vi "file list from temperatures file V2.vi"(6 "monotonic segments ON/OFF":bool=TRUE, 7 "action":T4(ring)=enum."update monotonic pieces", 9 "tfolder IN":T1={"tfolder path"=path "/snowfall/Users/arcadi/Desktop/Ultrasound/Experiment/YBCO_4/Round1/Sweep12/June_2011/062511/221.16400K_300_3100_001_062511.dat", "9folder path"=path "/snowfall/Users/arcadi/Desktop/Ultrasound/Experiment/YBCO_4/Round1/Sweep12/June_2011/062511/221.16400K_300_3100_001_062511.dat", "tfolder  -  file array"=[], "from index array"=[], "timestamp array"=[]}, 11 "tfolder file path  IN":path=path "/snowfall/Users/arcadi/Desktop/Ultrasound/Experiment/YBCO_4/Round1/Sweep12/June_2011/062511/221.16400K_300_3100_001_062511.dat") -> (0 "timestamp OUT":dbl[](array[numeric]), 1 "tfolder OUT":T1={"tfolder path"=path "/snowfall/Users/arcadi/Desktop/Ultrasound/Experiment/YBCO_4/Round1/Sweep12/June_2011/062511/221.16400K_300_3100_001_062511.dat", "9folder path"=path "/snowfall/Users/arcadi/Desktop/Ultrasound/Experiment/YBCO_4/Round1/Sweep12/June_2011/062511/221.16400K_300_3100_001_062511.dat", "tfolder  -  file array"=[], "from index array"=[], "timestamp array"=[]}, 2 "sweep path array OUT":T3[](array[typedef]), 3 "temperature OUT":dbl[](array[numeric]))   [LabVIEW 2010]
uses:
  sweep file name.ctl
  tfolder -- monotonic segment.ctl
  tfolder.ctl
panel:
  in  "tfolder - monotonic segment":T2
  in  "sweep file name":T3={"temperature"=0.0, "temperature str"="", "file path"=path "/snowfall/Users/arcadi/Desktop/Ultrasound/Experiment/YBCO_4/Round1/Sweep12/June_2011/062511/221.16400K_300_3100_001_062511.dat", "last mod"=timestamp(0 s since 1904-01-01), "file name str"="", "mod time(min)"=0.0, "file format"=enum.""}
  in  "file path OK":bool=TRUE
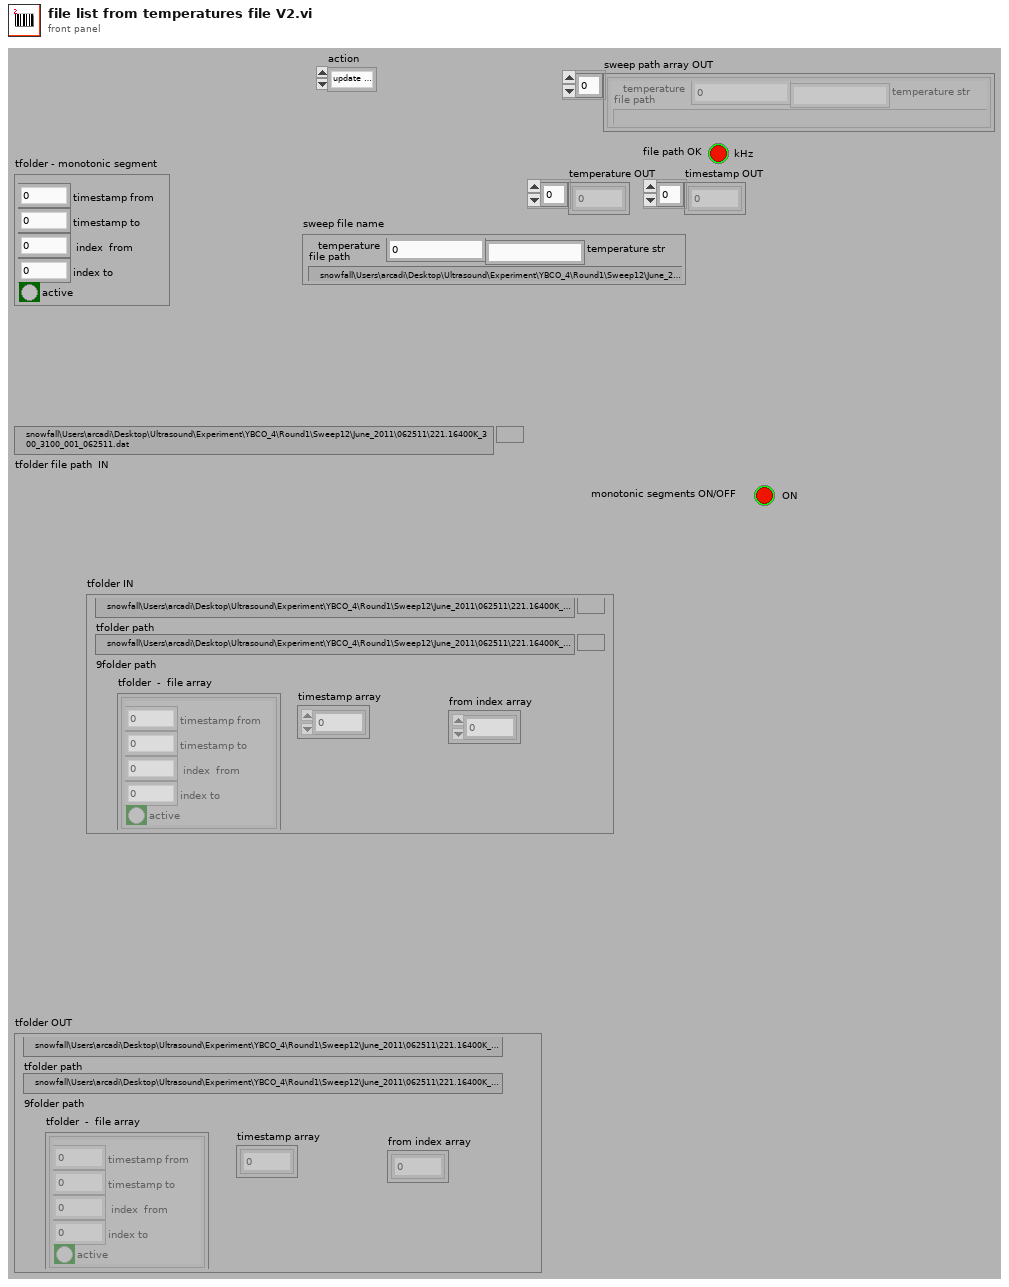
[diagram p1: front panel]
types:
  T1 = typedef "tfolder.ctl" = cluster{"tfolder path":path, "9folder path":path, "tfolder  -  file array":T2[], "from index array":i32[], "timestamp array":dbl[]}
  T2 = typedef "tfolder -- monotonic segment.ctl" = cluster{"timestamp from":dbl, "timestamp to":dbl, " index  from":i32, "index to":i32, "active":bool}
  T3 = typedef "sweep file name.ctl" = cluster{"temperature":dbl, "temperature str":string, "file path":path, "last mod":timestamp, "file name str":string, "mod time(min)":dbl, "file format":enum16{"", "ascii", "binary"}}
  T4 = enum16{"new", "update range", "update monotonic pieces", "init", "check", "reset", ""}
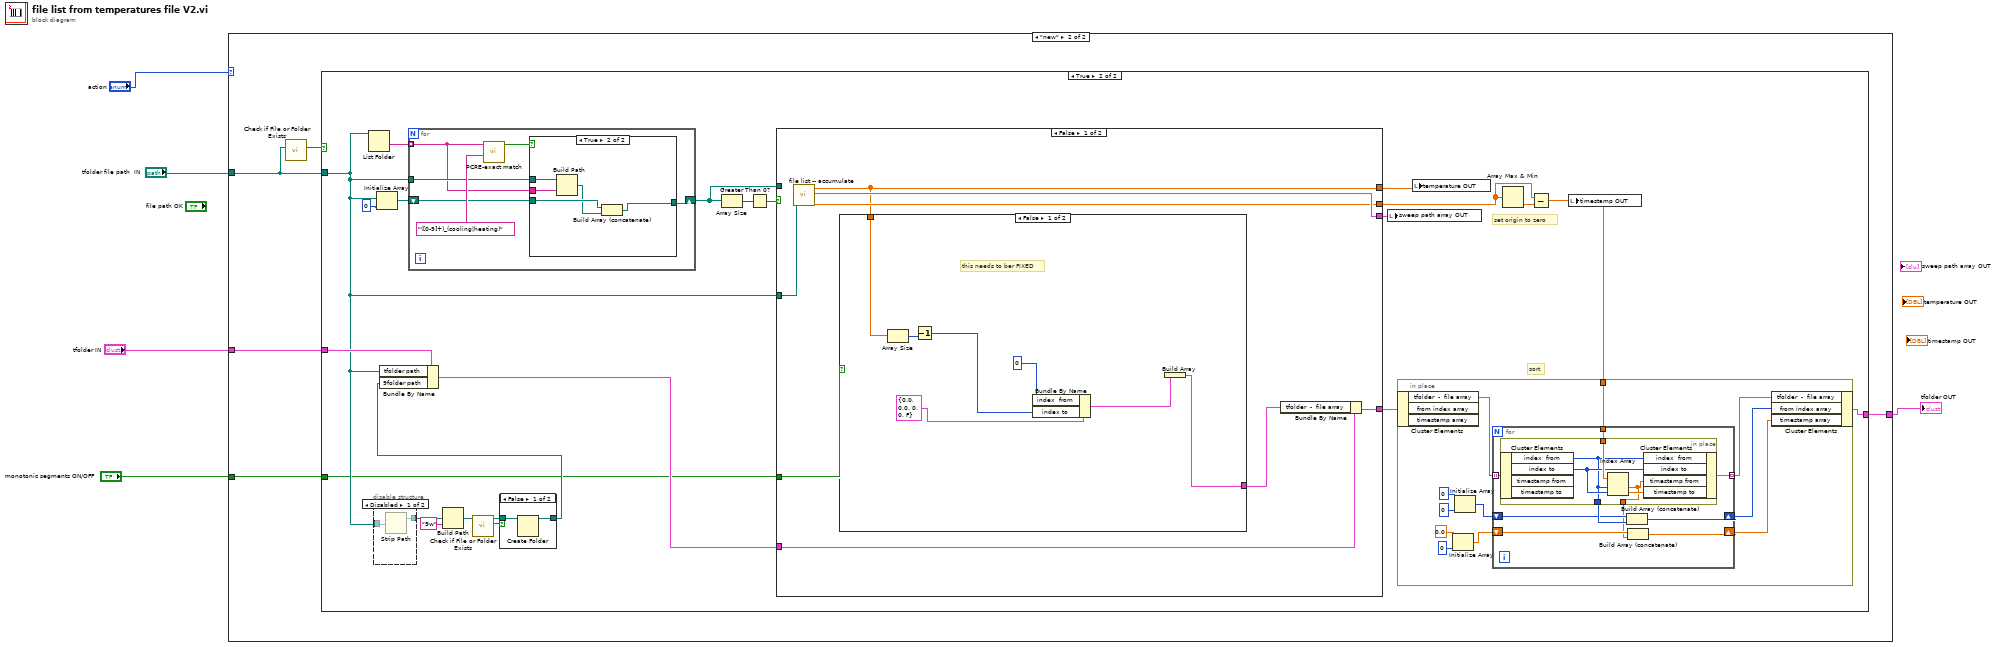
[diagram p0: block diagram]
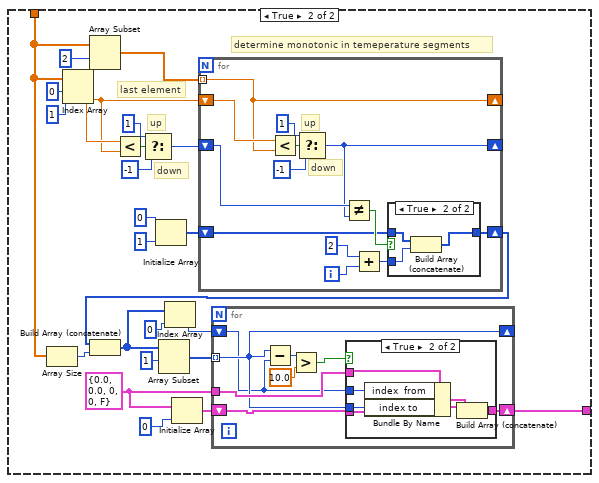
[diagram p6: hidden frame]
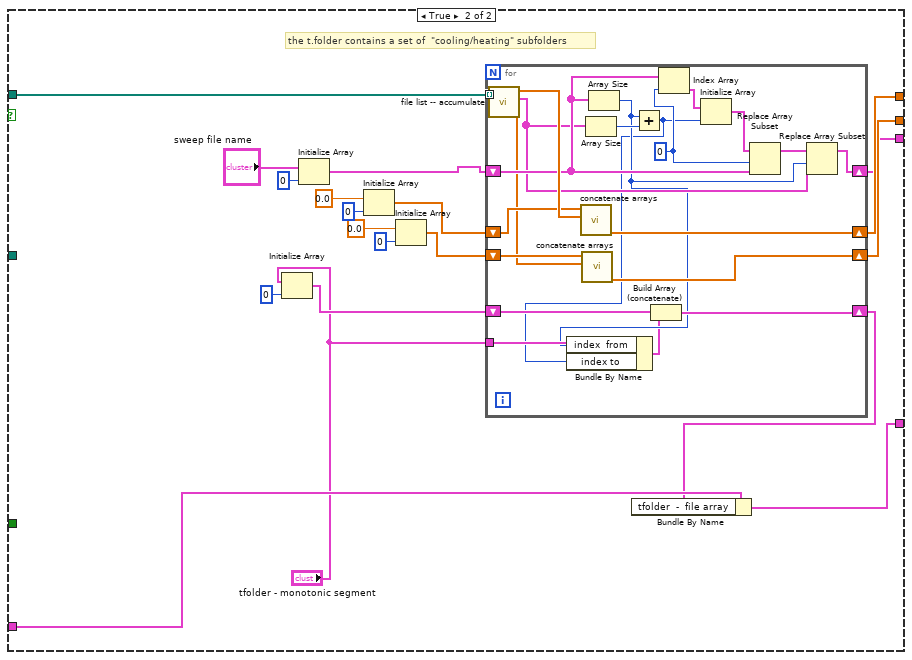
[diagram p9: hidden frame]
diagram:
  n1 = case shown="\"new\"" "action" {
    tunnel: "tfolder file path  IN" -> [_ w10]
    tunnel: "tfolder IN" -> [w6 w9]
    tunnel: [w6 w8] -> w2
    tunnel: "monotonic segments ON/OFF" -> [_ w7]
    frame "", Default {
    }
    frame "new" {
      n2 = call <vilib>:"Check if File or Folder Exists.vi"("path"=w10) -> ("file or folder exists?"=w11:bool)  [unwired: 8 in, 2 out]
      n3 = case shown="True" w11 {
        tunnel: w10 -> [_ w20]
        tunnel: w9 -> [w12 w29]
        tunnel: [w12 w15] -> w8
        tunnel: w7 -> [_ w13]
        frame False {
        }
        frame True {
          # "sort"
          # "set origin to zero"
          n4 = List Folder(path=w20) -> (folder names=w34:string[])  [unwired: 3 in, 3 out]
          n5 = disable-structure shown="Disabled" {
            disable-tunnel: [w65 w66] -> w28
            disable-tunnel: w20 -> [w64 w66]
            frame Disabled {
              n6 = Strip Path(path=w64) -> (stripped path=w65:path)  [unwired: 1 out]
            }
            frame Enabled {
            }
          }
          n7 = Initialize Array(w20, 0 ("dimension size")) -> (w33:path[])
          n8 = for {
            tunnel: w34 -> [w181] mode=indexing
            shift-right: [w179] -> w30
            shift-left: w33 -> [w180]
            tunnel: w20 -> [w182]
            n9 = call "PCRE-exact match.vi"("regular expression"="([0-9]+)_(cooling|heating)", "input string"=w181) -> ("exact match"=w183:bool)  [unwired: 8 in, 1 out]
            n10 = case shown="True" w183 {
              tunnel: w182 -> [_ w190]
              tunnel: w181 -> [_ w189]
              tunnel: w180 -> [w185 w188]
              tunnel: [w185 w186] -> w179
              frame False {
              }
              frame True {
                n11 = Build Path(base path=w190, name or relative path=w189) -> (appended path=w187:path)
                n12 = Build Array (concatenate)(w188, w187) -> (w186:path[])
              }
            }
          }
          n13 = Build Path(base path=w28, name or relative path="9w") -> (appended path=w26:path)
          n14 = call <vilib>:"Check if File or Folder Exists.vi"("path"=w26) -> ("file or folder exists?"=w25:bool, "dup path"=w24:path)  [unwired: 8 in, 1 out]
          n15 = case shown="False" w25 {
            tunnel: [w61 w63] -> w23
            tunnel: w24 -> [w62 w63]
            frame False {
              n16 = Create Folder(path (use dialog)=w62) -> (created path=w61:path)  [unwired: 2 in, 2 out]
            }
            frame True {
            }
          }
          n17 = Bundle By Name(cluster=w29, "tfolder path"=w20, "9folder path"=w23) -> (w21:T1)
          n18 = Array Size(array=w30) -> (size(s)=w32:i32)
          n19 = Greater Than 0?(x=w32) -> (x > 0?=w31:bool)
          n20 = case shown="False" w31 {
            tunnel: w30 -> [_ w157]
            tunnel: [w69 w156] -> w17
            tunnel: [w68 w155] -> w19
            tunnel: [w74 w154] -> w22
            tunnel: w21 -> [w72 w151]
            tunnel: [w71 w150] -> w16
            tunnel: w20 -> [w73 _]
            tunnel: w13 -> [w67 _]
            frame False {
              n21 = call "file list -- accumulate.vi"("file path"=w73) -> ("timestamp"=w69:dbl[], "sweep file name array"=w74:T3[], "temperatures"=w68:dbl[])  [unwired: 8 in]
              n22 = case shown="False" w67 {
                tunnel: [w75 w102] -> w70
                tunnel: w68 -> [w80 w82]
                frame False {
                  # "this needs to ber FIXED"
                  n23 = Array Size(array=w80) -> (size(s)=w79:i32)
                  n24 = Decrement(x=w79) -> (x-1=w77:i32)
                  n25 = Bundle By Name(cluster=T2 {"timestamp from"=0.0, "timestamp to"=0.0, " index  from"=0, "index to"=0, "active"=FALSE} ("monotonic segment"), "index  from"=0, "index to"=w77) -> (w81:T2)
                  n26 = Build Array(w81) -> (w75:T2[])
                }
                frame True {
                  w103 = T2 {"timestamp from"=0.0, "timestamp to"=0.0, " index  from"=0, "index to"=0, "active"=FALSE} ("monotonic segment")
                  # "determine monotonic in temeperature segments"
                  # "last element"
                  # "down"
                  # "up"
                  n27 = Array Size(array=w82) -> (size(s)=w84:i32)
                  n28 = Index Array(array=w82, index #1=0 ("dimension size"), index #2=1 ("dimension size")) -> (element #1=w95:dbl, element #2=w94:dbl)
                  n29 = Array Subset(array=w82, index=2 ("dimension size")) -> (w96:dbl[])  [unwired: 1 in]
                  n30 = Less?(x=w95, y=w94) -> (x < y?=w86:bool)
                  n31 = Select(t=1 ("dimension size"), s=w86, f=-1 ("dimension size")) -> (s? t:f=w91:i32)
                  n32 = Initialize Array(0 ("dimension size"), 1 ("dimension size")) -> (w101:i32[])
                  n33 = Initialize Array(w103, 0 ("dimension size")) -> (w104:T2[])
                  n34 = for {
                    shift-right: [w107] -> w85
                    shift-left: w101 -> [w109]
                    shift-right: [w115] -> _
                    shift-left: w94 -> [w116]
                    tunnel: w96 -> [w115] mode=indexing
                    shift-right: [w111] -> _
                    shift-left: w91 -> [w112]
                    i -> [w114]
                    # "down"
                    # "up"
                    n35 = Less?(x=w116, y=w115) -> (x < y?=w119:bool)
                    n36 = Select(t=1 ("dimension size"), s=w119, f=-1 ("dimension size")) -> (s? t:f=w111:i32)
                    n37 = Not Equal?(x=w112, y=w111) -> (x != y?=w110:bool)
                    n38 = Add(x=2, y=w114) -> (x+y=w108:i32)
                    n39 = case shown="True" w110 {
                      tunnel: w109 -> [w120 w123]
                      tunnel: w108 -> [_ w122]
                      tunnel: [w120 w121] -> w107
                      frame False {
                      }
                      frame True {
                        n40 = Build Array (concatenate)(w123, w122) -> (w121:i32[])
                      }
                    }
                  }
                  n41 = Build Array (concatenate)(w85, w84) -> (w83:i32[])
                  n42 = Array Subset(array=w83, index=1 ("dimension size")) -> (w87:i32[])  [unwired: 1 in]
                  n43 = Index Array(array=w83, index=0 ("dimension size")) -> (element=w89:i32)
                  n44 = for {
                    shift-right: [w130] -> w102
                    shift-left: w104 -> [w131]
                    tunnel: w103 -> [w129]
                    shift-right: [w126] -> _
                    shift-left: w89 -> [w125]
                    tunnel: w87 -> [w126] mode=indexing
                    n45 = Subtract(x=w126, y=w125) -> (x-y=w128:i32)
                    n46 = Greater?(x=w128, y=10.0) -> (0:w124:bool)
                    n47 = case shown="True" w124 {
                      tunnel: w131 -> [w132 w138]
                      tunnel: [w132 w137] -> w130
                      tunnel: w129 -> [_ w135]
                      tunnel: w126 -> [_ w134]
                      tunnel: w125 -> [_ w133]
                      frame False {
                      }
                      frame True {
                        n48 = Bundle By Name(cluster=w135, "index  from"=w133, "index to"=w134) -> (w136:T2)
                        n49 = Build Array (concatenate)(w138, w136) -> (w137:T2[])
                      }
                    }
                  }
                }
              }
              n50 = Bundle By Name(cluster=w72, "tfolder  -  file array"=w70) -> (w71:T1)
            }
            frame True {
              # "the t.folder contains a set of  \"cooling/heating\" subfolders"
              n51 = Initialize Array("tfolder - monotonic segment", 0 ("dimension size")) -> (w152:T2[])
              n52 = Initialize Array("sweep file name", 0 ("dimension size")) -> (w143:T3[])
              n53 = Initialize Array(0.0 ("dimension size"), 0 ("dimension size")) -> (w142:dbl[])
              n54 = Initialize Array(0.0 ("dimension size"), 0 ("dimension size")) -> (w141:dbl[])
              n55 = for {
                tunnel: w157 -> [w178] mode=indexing
                shift-right: [w167] -> w154
                shift-left: w143 -> [w169]
                shift-right: [w172] -> w155
                shift-left: w142 -> [w173]
                shift-right: [w164] -> w156
                shift-left: w141 -> [w166]
                shift-right: [w162] -> w139
                shift-left: w152 -> [w163]
                tunnel: "tfolder - monotonic segment" -> [w161]
                w171 = 0 ("dimension size")
                n56 = call "file list -- accumulate.vi"("file path"=w178) -> ("timestamp"=w165:dbl[], "sweep file name array"=w168:T3[], "temperatures"=w174:dbl[])  [unwired: 8 in]
                n57 = call "concatenate arrays.vi"("Array 2"=w174, "Array 1"=w173) -> ("output array 2"=w172:dbl[])  [unwired: 9 in]
                n58 = call "concatenate arrays.vi"("Array 2"=w165, "Array 1"=w166) -> ("output array 2"=w164:dbl[])  [unwired: 9 in]
                n59 = Array Size(array=w168) -> (size(s)=w177:i32)
                n60 = Array Size(array=w169) -> (size(s)=w160:i32)
                n61 = Add(x=w160, y=w177) -> (x+y=w159:i32)
                n62 = Bundle By Name(cluster=w161, "index  from"=w160, "index to"=w159) -> (w158:T2)
                n63 = Build Array (concatenate)(w163, w158) -> (w162:T2[])
                n64 = Index Array(array=w169, index=w171) -> (element=w170:T3)
                n65 = Initialize Array(w170, w159) -> (w176:T3[])
                n66 = Replace Array Subset(array=w176, new element=w169, index=w171) -> (w175:T3[])
                n67 = Replace Array Subset(array=w175, new element=w168, index=w160) -> (w167:T3[])
              }
              n68 = Bundle By Name(cluster=w151, "tfolder  -  file array"=w139) -> (w150:T1)
            }
          }
          n69 = local write "sweep path array OUT"(w22) -> ()
          n70 = local write "temperature OUT"(w19) -> ()
          n71 = Array Max & Min(array=w17) -> (min value=w18:dbl)  [unwired: 3 out]
          n72 = Subtract(x=w17, y=w18) -> (x-y=w14:dbl[])
          n73 = in-place {
            in-place-border: w14 -> [w45]
            n74 = in-place-cluster #1(w16) -> ("tfolder  -  file array"=w46:T2[])  [unwired: 2 out]
            n75 = Initialize Array(0.0 ("dimension size"), 0 ("dimension size")) -> (w39:dbl[])
            n76 = Initialize Array(0 ("dimension size"), 0 ("dimension size")) -> (w38:i32[])
            n77 = for {
              tunnel: w46 -> [w55] mode=indexing
              tunnel: w45 -> [w54]
              tunnel: [w53] -> w44 mode=indexing
              shift-right: [w48] -> w36
              shift-left: w38 -> [w50]
              shift-right: [w49] -> w37
              shift-left: w39 -> [w52]
              n78 = in-place {
                in-place-border: w54 -> [w60]
                in-place-border: [w57] -> w51
                in-place-border: [w56] -> w47
                n79 = in-place-cluster #2(w55) -> ("index  from"=w57:i32, "index to"=w58:i32)  [unwired: 2 out]
                n80 = Index Array(array=w60, index #1=w57, index #2=w58) -> (element #1=w56:dbl, element #2=w59:dbl)
                n81 = in-place-cluster #2("index  from"=w57, "index to"=w58, "timestamp from"=w56, "timestamp to"=w59) -> (w53:T2)
              }
              n82 = Build Array (concatenate)(w50, w51) -> (w48:i32[])
              n83 = Build Array (concatenate)(w52, w47) -> (w49:dbl[])
            }
            n84 = in-place-cluster #1("tfolder  -  file array"=w44, "from index array"=w36, "timestamp array"=w37) -> (w15:T1)
          }
          n85 = local write "timestamp OUT"(w14) -> ()
        }
      }
    }
  }
  "tfolder OUT" <- w2
